vi "Enable UI.vi"(8 "error in (no error)":errorcluster, 11 "Measurement UI in":refnum<class "Measurement UI.lvclass">) -> (0 "error out":errorcluster, 3 "Measurement UI out":refnum<class "Measurement UI.lvclass">)   [LabVIEW 2015, in "Measurement UI.lvlib" / "Measurement UI.lvclass"]
uses:
  Measurement UI.lvclass
  Measurement UI.lvclass/Measurement UI.ctl
  Accessors/Read Load New Measurement.vi
  Accessors/Read Measurement.vi
  Accessors/Read Show FP_.vi
  User Interface/UI.lvclass
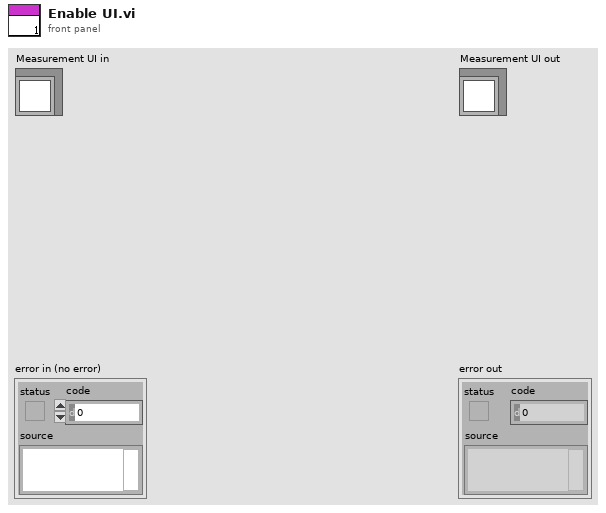
[diagram p1: front panel]
types:
  T1 = enum8{"Enabled", "Disabled", "Disabled and Grayed Out"}
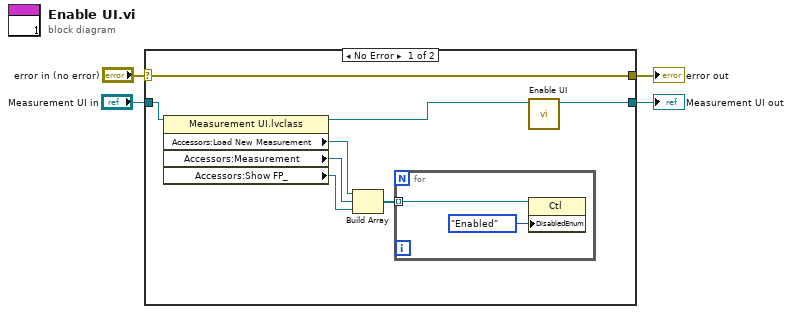
[diagram p0: block diagram]
diagram:
  n1 = case shown="No Error" "error in (no error)" {
    selector: "error in (no error)" -> [w12 w16]
    tunnel: [w12 w16] -> w3
    tunnel: [w6 w15] -> w1
    tunnel: "Measurement UI in" -> [w8 w15]
    frame No Error {
      n2 = property class="Measurement UI.lvclass"(reference=w8) -> (reference out=w7:refnum<class "Measurement UI.lvclass">, "Accessors:Load New Measurement"=w5:refnum<vi>, "Accessors:Measurement"=w9:refnum<vi>, "Accessors:Show FP_"=w10:refnum<vi>)  [unwired: 1 in, 1 out]
      n3 = Build Array(w5, w9, w10) -> (w11:refnum<vi>[])
      n4 = for {
        tunnel: w11 -> [w14] mode=indexing
        n5 = property class="Ctl"(reference=w14, "DisabledEnum"=T1."Enabled" ("Disabled")) -> ()  [unwired: 1 in, 2 out]
      }
      n6 = call-parent "Enable UI.vi"("UI in"=w7) -> ("UI out"=w6:refnum<class "Measurement UI.lvclass">)  [unwired: 9 in, 1 out]
    }
    frame Error {
    }
  }
  "error out" <- w3
  "Measurement UI out" <- w1
